vi "Generate Report Get Data to Modify.vi"(4 "error in (no error)":errorcluster, 5 "ms timeout (-1)":i32=-1, 7 "report in":T2) -> (0 "error out":errorcluster, 1 "timed out":bool, 2 "data":T1, 3 "report out":T2)   [LabVIEW 2012, in "NISH Report.lvlib"]
doc: "This VI returns the data associated with the <B>Generate Report</B> object reference and places a lock on the object.\n\nIf the object is currently locked for modification by another method, <B>timeout</B> specifies how long the VI should wait to receive access to the object. The default value waits until the object becomes available.\n\nIf the object does not become available for modification during <B>timeout</B> milliseconds, <B>timed out</B> will return TRUE.\n\nIf, and only if, you successfully locked the object's data for modification (i.e. <B>timed out</B> returned FALSE), you must use the <B>Generate Report Set Modified Data</B> VI to set the object's data and release the lock.\n\n[GOOP 1.0/1.0]"
uses:
  <resource>/importtools/NISH Report/NISH Report.lvlib
  <resource>/importtools/NISH Report/Generate Report Data Members.ctl
  <resource>/importtools/NISH Report/Generate Report Object Reference.ctl
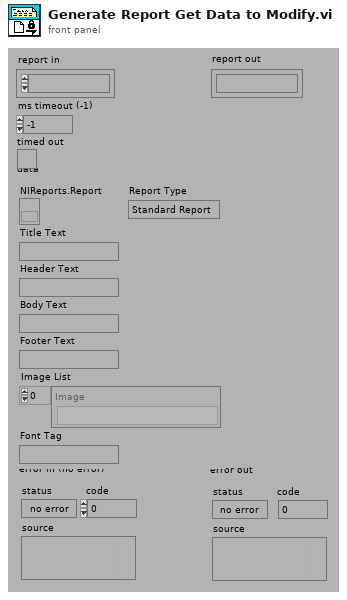
[diagram p1: front panel]
types:
  T1 = typedef "NISH Report.lvlib/Generate Report Data Members.ctl" = cluster{"Title Text":string, "Header Text":string, "Body Text":string, "Footer Text":string, "Image List":string[], "NIReports.Report":refnum<k7>, "Report Type":enum16{"Standard Report", "HTML"}, "Font Tag":string}
  T2 = typedef "NISH Report.lvlib/Generate Report Object Reference.ctl" = refnum<k1>
  T3 = enum16{"Create", "GetCopy", "GetModify", "Set", "Destroy", "Create Static", "Get All Refs", "Reset", "Get Statistics"}
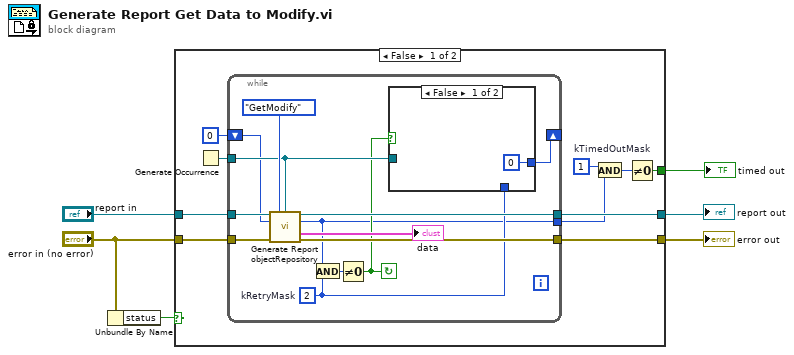
[diagram p0: block diagram]
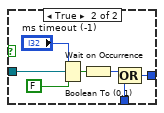
[diagram p2: hidden frame]
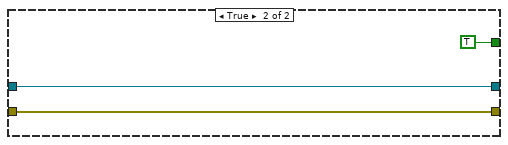
[diagram p3: hidden frame]
diagram:
  n1 = Unbundle By Name("error in (no error)") -> ("status"=w6:bool)
  n2 = case shown="False" w6 {
    tunnel: "error in (no error)" -> [w16 w40]
    tunnel: [w13 w40] -> w4
    tunnel: "report in" -> [w15 w39]
    tunnel: [w14 w39] -> w2
    tunnel: [w7 TRUE] -> w1
    frame False {
      w9 = 1  # kTimedOutMask
      n3 = Generate Occurrence() -> (w11:refnum<k4>)
      n4 = while {
        tunnel: [w17] -> w8
        tunnel: w11 -> [w23]
        shift-left: 0 -> [w21]
        shift-right: [w18] -> _
        tunnel: [w28] -> w13
        tunnel: [w29] -> w14
        tunnel: w15 -> [w27]
        tunnel: w16 -> [w26]
        stop <- w20 continue-if-true
        w19 = 2  # kRetryMask
        n5 = call <resource>:"Generate Report objectRepository.vi"("reference in"=w27, "method"=T3."GetModify", "occurrence"=w23, "flags in"=w21, "error in (no error)"=w26) -> ("reference out"=w29:T2, "flags out"=w17:i32, "classDataOut"=→"data":T1, "error out"=w28:errorcluster)  [unwired: 4 in, 3 out]
        n6 = And(x=w17, y=w19) -> (x .and. y?=w22:i32)
        n7 = Not Equal To 0?(x=w22) -> (x != 0?=w20:bool)
        n8 = case shown="False" w20 {
          tunnel: w23 -> [_ w35]
          tunnel: w19 -> [_ w32]
          tunnel: [0 w31] -> w18
          frame False {
          }
          frame True {
            n9 = Wait on Occurrence(1:FALSE ("ignore previous (T)"), 2:w35, 3:"ms timeout (-1)") -> (0:w33:bool)
            n10 = Boolean To (0,1)(Boolean=w33) -> (0, 1=w34:i16)
            n11 = Compound Arithmetic op=OR(w34, w32) -> (w31:i32)
          }
        }
      }
      n12 = And(x=w9, y=w8) -> (x .and. y?=w10:i32)
      n13 = Not Equal To 0?(x=w10) -> (x != 0?=w7:bool)
    }
    frame True {
    }
  }
  "error out" <- w4
  "report out" <- w2
  "timed out" <- w1
